vi "DispBallTacticVSS.vi"(6 "State":enum16{"BallDispPos", "Exit"}(ring), 9 "Game in":refnum<class "Game.lvclass">, 10 "Robot":refnum<class "Robot.lvclass">, 11 "DispBallTacticVSS in":refnum<class "DispBallTacticVSS.lvclass">) -> (2 "Robot out":refnum<class "Robot.lvclass">, 3 "DispBallTacticVSS out":refnum<class "DispBallTacticVSS.lvclass">)   [LabVIEW 2023, in "DispBallTacticVSS.lvclass"]
uses:
  DispBallTacticVSS.lvclass
  Robot_class/Robot.lvclass
  Game_class/Game.lvclass
  Robot_class/tactics.ctl
  Tactic_class/Tactic.lvclass/Tactic.ctl
  Robot_class/Robot.lvclass/Robot.ctl
  Tactic_class/Read Skillbook.vi
  Robot_class/Write tactic.vi
  Skillbook_class/Skillbook.lvclass
  KickSkillVSS_class/KickSkillVSS.lvclass
  PenaltyPosSkillVSS_class/PenaltyPosSkillVSS.lvclass
  BallDispPosSkillVSS_class/BallDispPosSkillVSS.lvclass
  BallToGoalSkillVSS_class/BallToGoalSkillVSS.lvclass
  GoToBallSkillVSS_class/GoToBallSkillVSS.lvclass
  DefBallPosSkillVSS_class/DefBallPosSkillVSS.lvclass
  HaltSkill_class/HaltSkill.lvclass
  KeeperDefPosSkillVSS_class/KeeperDefPosSkillVSS.lvclass
  GoToBallKeeperSkillVSS_class/GoToBallKeeperSkillVSS.lvclass
  RotateWallSkillVSS_class/RotateWallSkillVSS.lvclass
panel:
  out "x .or. y?":bool
  out "error out 2":errorcluster
  in  "error in (no error) 2":errorcluster
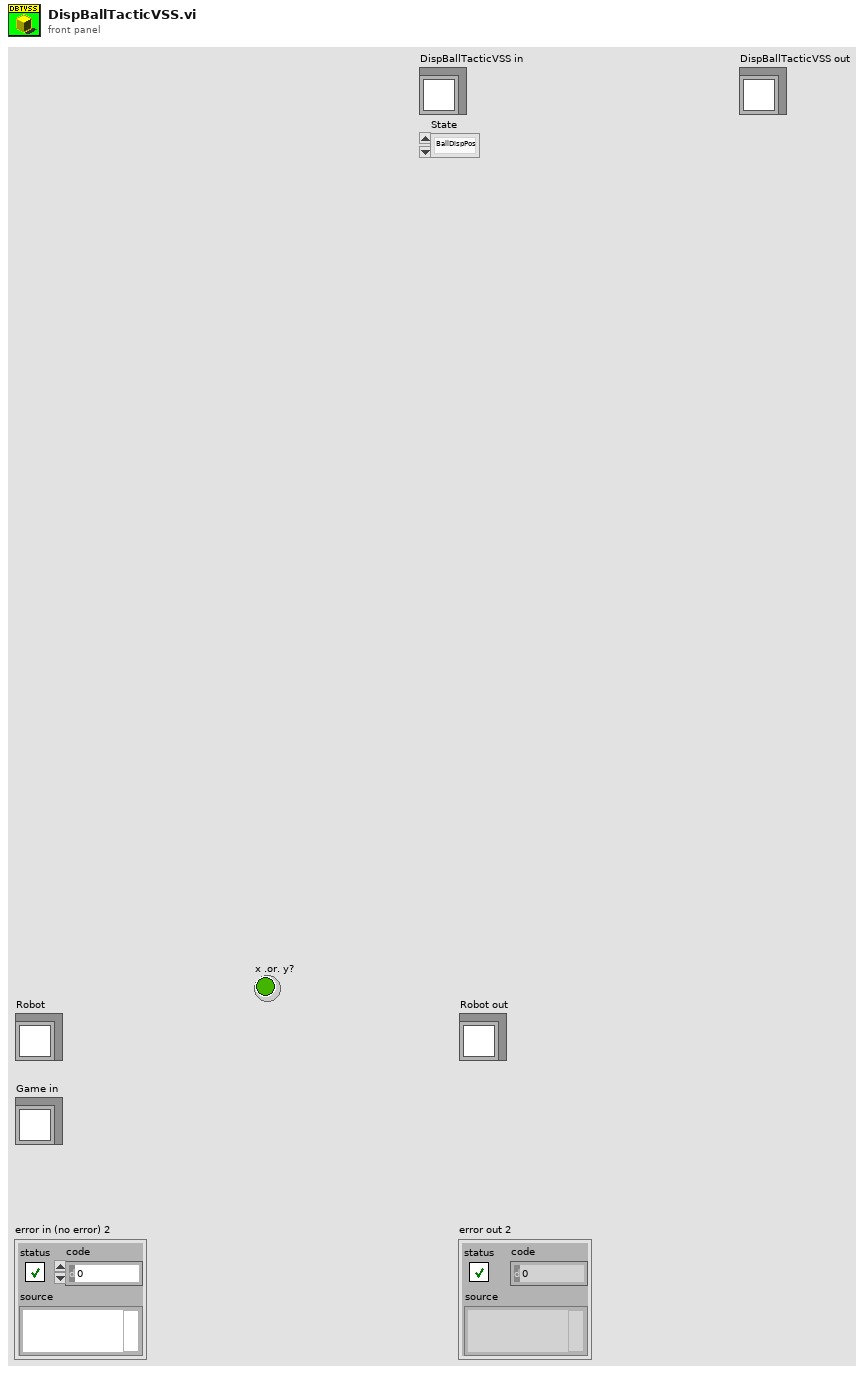
[diagram p1: front panel]
types:
  T1 = typedef "tactics.ctl" = enum16{"ReceivePassInFuturePoint", "Roller", "PrepareRollToPassRollerGoTo", "PrepareRollToPassReceiverGoTo", "WaitRoll", "PositionToRoll", "PenaltyAttacker", "PassObserver", "PenaltyDefense", "TableReceiverTactic", "Test", "DefendGoal", "Marker", "FollowAttacker", "DefendArea", "Shoot", "AttackerAimGoal", "AttackerBallOutOfField", "AttackerBlock", "AttackerStop", "Duelist", "Halt", "ZigZag", "GoTo", "Timeout", "KickToPassReceiver", "PositionToReceivePass", "DefendAreaVSS", "DefendGoalVSS", "KickVSS", "AttackVSS", "DispBallVSS", "PenaltyAttackVSS", "WaitPass"}
  T2 = cluster{"KickSkillVSS":refnum<class "KickSkillVSS.lvclass">, "PenaltyPosSkillVSS":refnum<class "PenaltyPosSkillVSS.lvclass">, "BallDispPosSkillVSS":refnum<class "BallDispPosSkillVSS.lvclass">, "BallToGoalSkillVSS":refnum<class "BallToGoalSkillVSS.lvclass">, "GoToBallSkillVSS":refnum<class "GoToBallSkillVSS.lvclass">, "DefBallPosSkillVSS":refnum<class "DefBallPosSkillVSS.lvclass">, "HaltSkill":refnum<class "HaltSkill.lvclass">, "KeeperDefPosSkillVSS":refnum<class "KeeperDefPosSkillVSS.lvclass">, "GoToBallKeeperSkillVSS":refnum<class "GoToBallKeeperSkillVSS.lvclass">, "RotateWallSkillVSS":refnum<class "RotateWallSkillVSS.lvclass">}
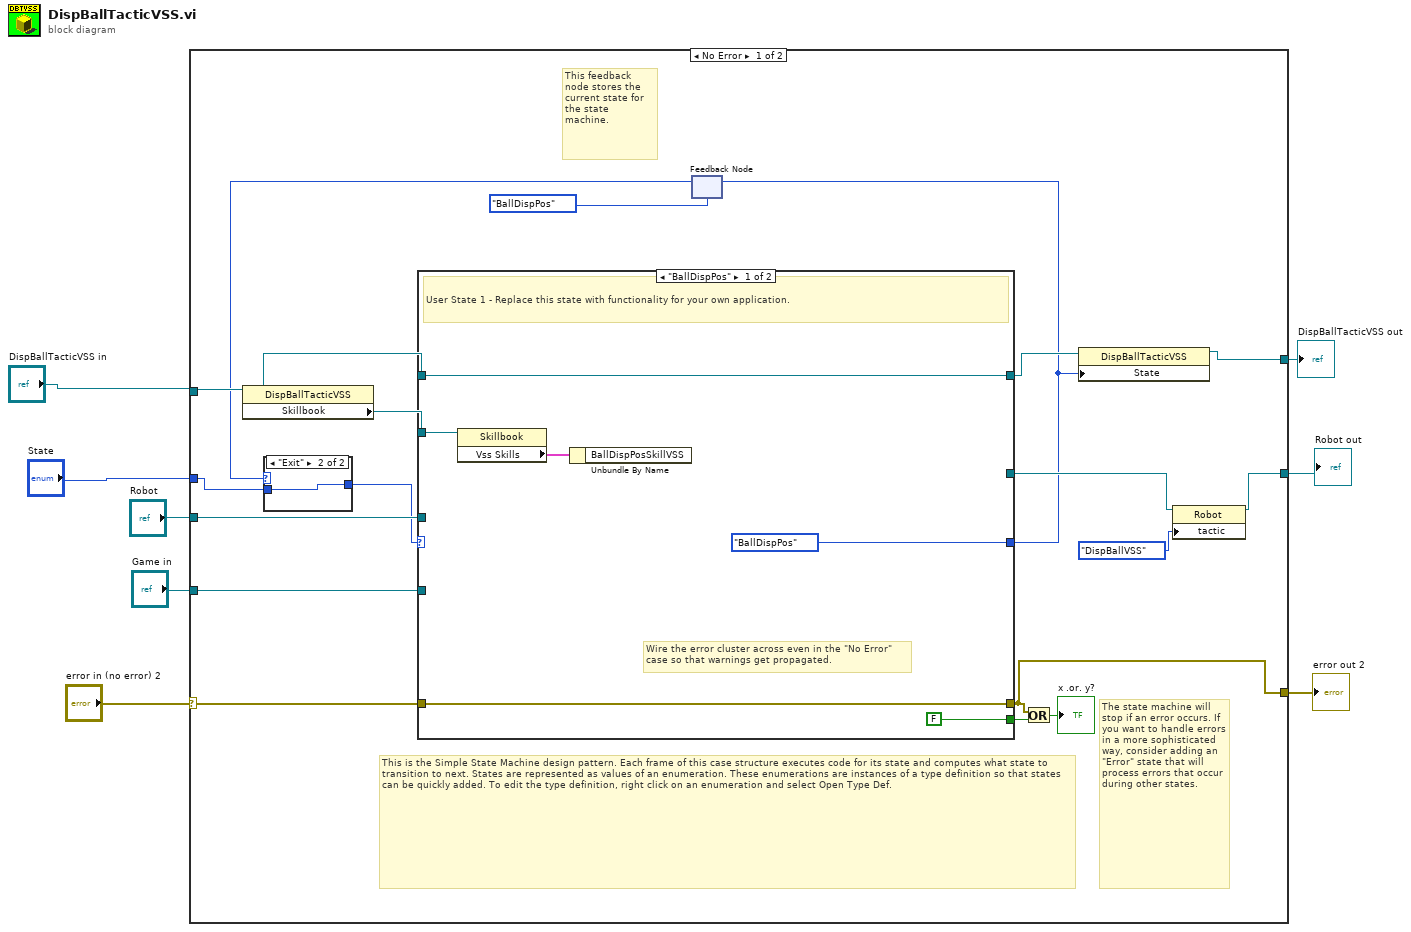
[diagram p0: block diagram]
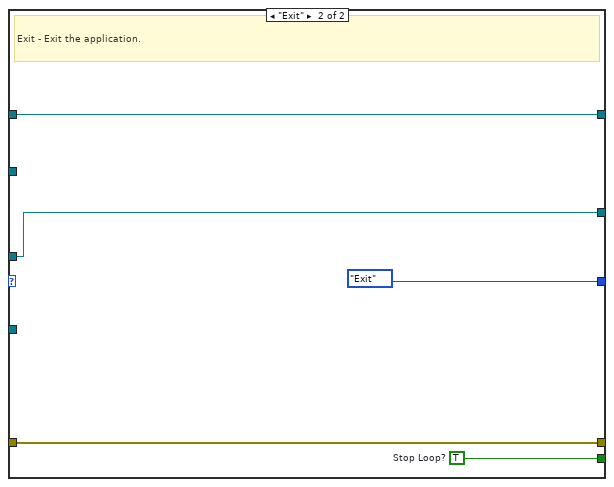
[diagram p3: hidden frame]
diagram:
  n1 = case shown="No Error" "error in (no error) 2" {
    selector: "error in (no error) 2" -> [w20 w42]
    tunnel: [w19 w42] -> w7
    tunnel: [w9 w41] -> w2
    tunnel: "DispBallTacticVSS in" -> [w23 w41]
    tunnel: "Robot" -> [w22 w40]
    tunnel: "Game in" -> [w21 _]
    tunnel: [w13 w40] -> w4
    tunnel: "State" -> [w16 _]
    frame No Error {
      # "The state machine will stop if an error occurs. If you want to handle errors in a more sophisticated way, consider adding an \"Error\" state that will process errors that occur during other states."
      # "This feedback node stores the current state for the state machine."
      # "This is the Simple State Machine design pattern. Each frame of this case structure executes code for its state and computes what state to transition to next. States are represented as values of an enumeration. These enumerations are instances of a type definition so that states can be quickly added. To edit the type definition, right click on an enumeration and select Open Type Def."
      # "Wire the error cluster across even in the \"No Error\"\ncase so that warnings get propagated."
      n2 = property class="DispBallTacticVSS"(reference=w23) -> ("Skillbook"=w24:refnum<class "Skillbook.lvclass">)  [unwired: 1 in, 2 out]
      n3 = feedback #1(enum16{"BallDispPos", "Exit"}."BallDispPos" ("State")) -> (w18:enum16{"BallDispPos", "Exit"})
      n4 = case shown="\"Exit\"" w18 {
        selector: w18 -> [w27 _]
        tunnel: [w27 w28] -> w17
        tunnel: w16 -> [_ w28]
        frame "BallDispPos" {
        }
        frame "Exit" {
        }
      }
      n5 = case shown="\"BallDispPos\"" w17 {
        tunnel: [enum16{"BallDispPos", "Exit"}."BallDispPos" ("State") enum16{"BallDispPos", "Exit"}."Exit" ("State")] -> w11
        tunnel: [FALSE ("Stop Loop?") w39] -> w26
        tunnel: w24 -> [w33 _]
        tunnel: w22 -> [_ w38]
        tunnel: [_ w38] -> w14
        tunnel: [w32 w37] -> w12
        tunnel: w23 -> [w32 w37]
        tunnel: w21 -> [_ _]
        tunnel: [w31 w36] -> w19
        tunnel: w20 -> [w31 w36]
        frame "BallDispPos" {
          # "User State 1 - Replace this state with functionality for your own application."
          n6 = property class="Skillbook"(reference=w33) -> ("Vss Skills"=w29:T2)  [unwired: 1 in, 2 out]
          n7 = Unbundle By Name(w29) -> ()  [unwired: 1 out]
        }
        frame "Exit" {
          w39 = TRUE  # Stop Loop?
          # "Exit - Exit the application."
        }
      }
      n8 = feedback-in #1(w11) -> ()
      n9 = Or(x=w19, y=w26) -> (x .or. y?=→"x .or. y?":bool)
      n10 = property class="DispBallTacticVSS"(reference=w12, "State"=w11) -> (reference out=w9:refnum<class "DispBallTacticVSS.lvclass">)  [unwired: 1 in, 1 out]
      n11 = property class="Robot"(reference=w14, "tactic"=tactics."DispBallVSS") -> (reference out=w13:refnum<class "Robot.lvclass">)  [unwired: 1 in, 1 out]
    }
    frame Error {
    }
  }
  "error out 2" <- w7
  "Robot out" <- w4
  "DispBallTacticVSS out" <- w2
